vi "_Read.vi"(8 "error in (no error)":errorcluster, 11 "Lockin SR830 in":refnum<class "Lockin SR830.lvclass">) -> (0 "error out":errorcluster, 2 "4 Data Points":dbl[](array[numeric]), 3 "Lockin SR830 out":refnum<class "Lockin SR830.lvclass">)   [LabVIEW 2009, in "Lockin SR830.lvclass"]
uses:
  Lockin SR830.lvclass
  <vilib>/regexp/Match Regular Expression.xnode
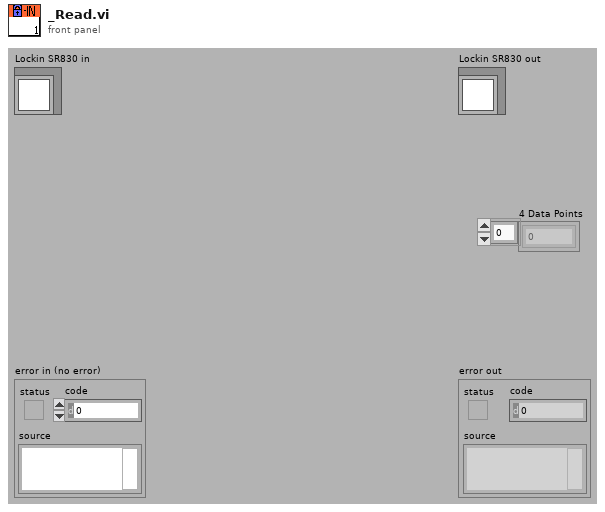
[diagram p1: front panel]
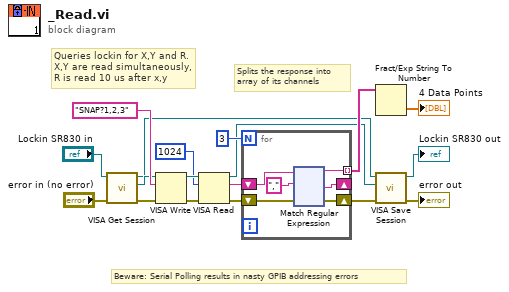
[diagram p0: block diagram]
diagram:
  # "Beware: Serial Polling results in nasty GPIB addressing errors"
  # "Queries lockin for X,Y and R.\nX,Y are read simultaneously, \nR is read 10 us after x,y"
  # "Splits the response into\narray of its channels"
  n1 = call-dynamic "VISA Get Session.vi"("error in (no error)"="error in (no error)", "Instrument.lvclass in"="Lockin SR830 in") -> ("error out"=w3:errorcluster, "VISA Resource Name"=w5:refnum<visa-resource-name>, "Instrument.lvclass out"=w4:refnum<class "Lockin SR830.lvclass">)  [unwired: 7 out]
  n2 = VISA Write(VISA resource name=w5, write buffer="SNAP?1,2,3", error in (no error)=w3) -> (VISA resource name out=w8:refnum<visa-resource-name>, error out=w2:errorcluster)  [unwired: 1 out]
  n3 = VISA Read(VISA resource name=w8, byte count=1024, error in (no error)=w2) -> (VISA resource name out=w7:refnum<visa-resource-name>, read buffer=w11:string, error out=w10:errorcluster)  [unwired: 1 out]
  n4 = for {
    N: 3 -> [_]
    tunnel: [w23] -> w14 mode=indexing
    shift-right: [w22] -> _
    shift-left: w11 -> [w21]
    shift-right: [w19] -> w6
    shift-left: w10 -> [w20]
    n5 = xnode "Match Regular Expression"("input string"=w21, "regular expression"=",", "error in"=w20) -> ("before match"=w23:string, "after match"=w22:string, "error out"=w19:errorcluster)  [unwired: 3 in, 2 out]
  }
  n6 = Fract/Exp String To Number(string=w14) -> (number=→"4 Data Points":dbl[])  [unwired: 3 in, 1 out]
  n7 = call-dynamic "VISA Save Session.vi"("error in (no error)"=w6, "VISA Resource Name"=w7, "Instrument.lvclass in"=w4) -> ("error out"=→"error out":errorcluster, "Instrument.lvclass out"=→"Lockin SR830 out":refnum<class "Lockin SR830.lvclass">)  [unwired: 7 out]
